vi "Read_data_from_saved_exp.vi"(10 "Path of file":path) -> (0 "Comments":string, 1 "Time Delays":dbl[](array[numeric]), 2 "Wavelengths":dbl[](array[numeric]), 3 "Data":dbl[][](array[numeric]), 4 "data raw":i32[][][][](array[numeric]), 5 "Number of points":i32, 6 "Step":dbl, 7 "Zero time delay":dbl, 8 "error out":errorcluster)   [LabVIEW 2015]
uses:
  <vilib>/Utility/file.llb/Read Delimited Spreadsheet (DBL).vi
  <vilib>/zip/NI_Unzip.lvlib
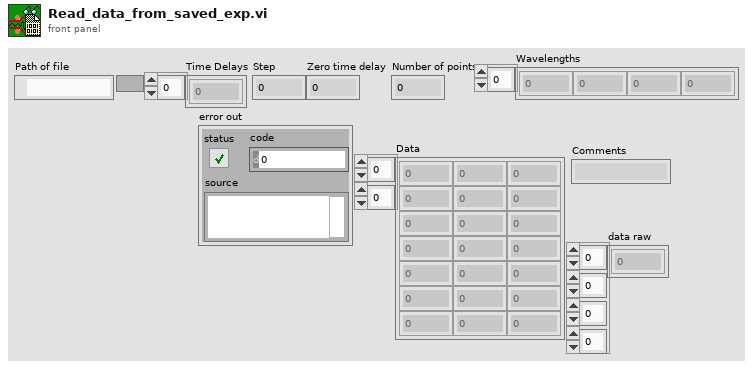
[diagram p1: front panel]
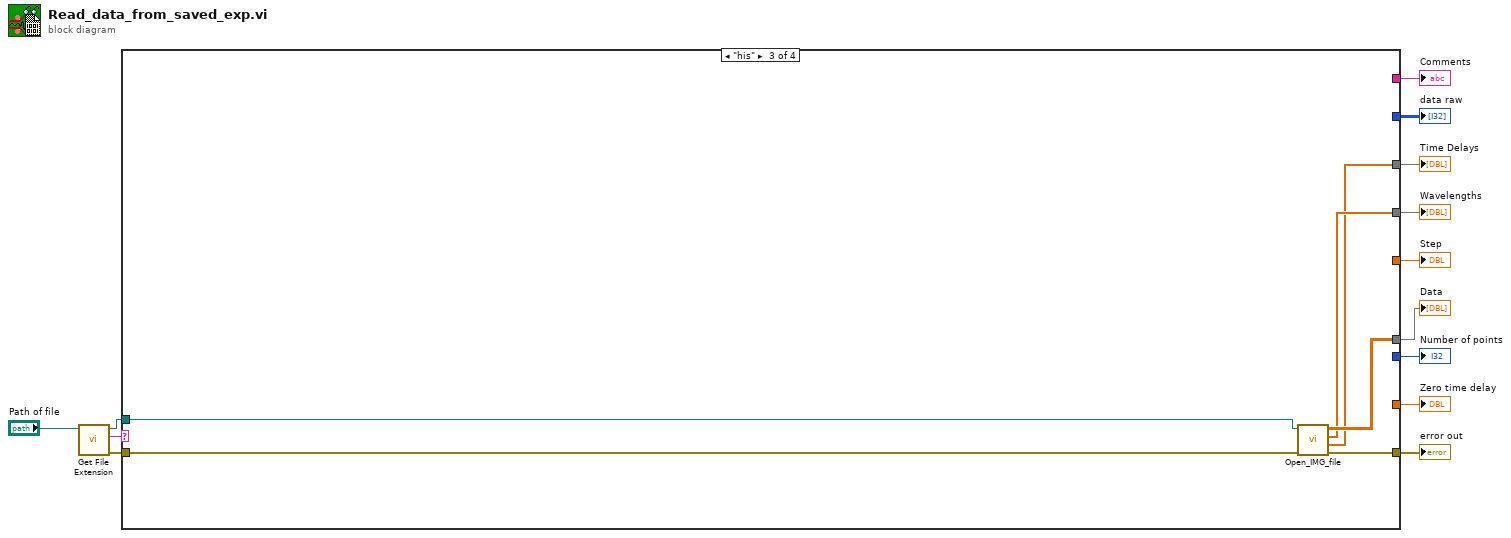
[diagram p0: block diagram]
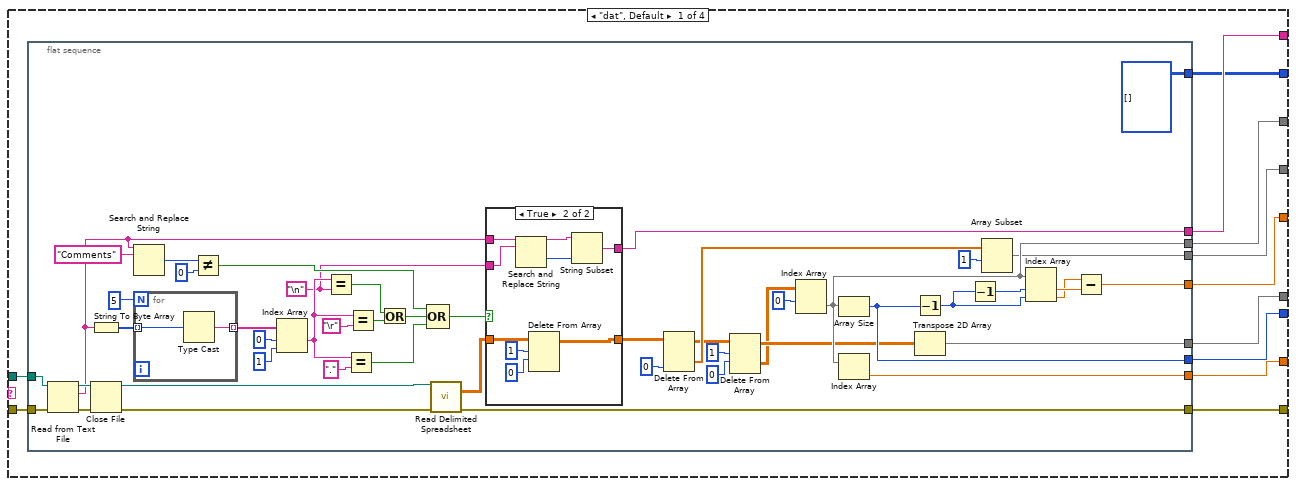
[diagram p2: hidden frame]
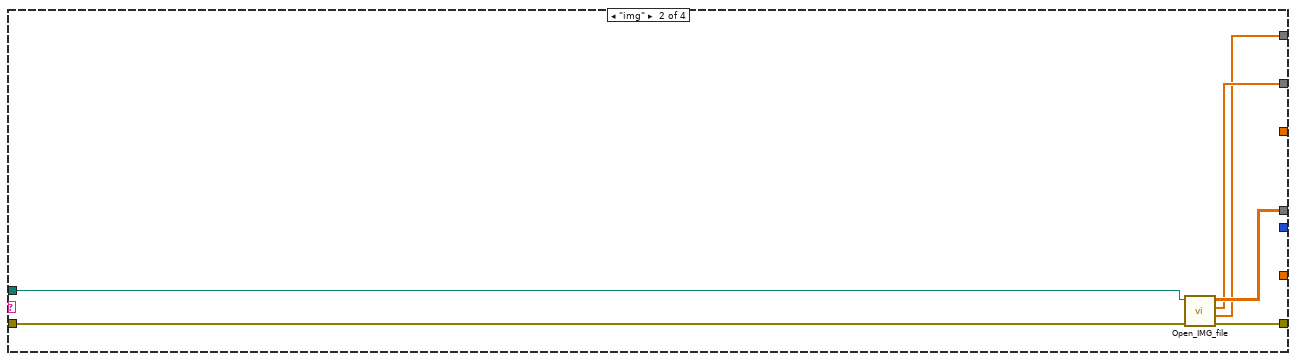
[diagram p4: hidden frame]
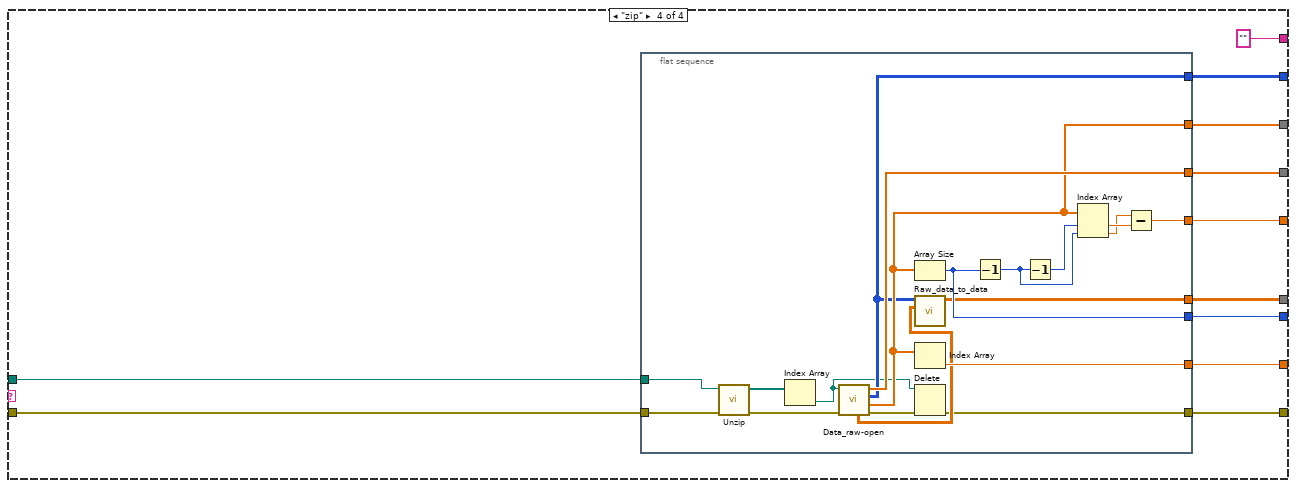
[diagram p5: hidden frame]
diagram:
  n1 = call <vilib>:"Get File Extension.vi"("file"="Path of file") -> ("error out"=w3:errorcluster, "lowercase file extension"=w4:string, "dup file"=w6:path)  [unwired: 6 in, 2 out]
  n2 = case shown="\"his\"" w4 {
    tunnel: [w24 _ _ w108] -> w13
    tunnel: [w23 w88 w94 w107] -> w12
    tunnel: [w22 w86 w92 w106] -> w11
    tunnel: [w21 _ _ w105] -> w10
    tunnel: [w20 _ _ w104] -> w9
    tunnel: [w19 w87 w93 w103] -> w8
    tunnel: w6 -> [w18 w91 w97 w102]
    tunnel: [w17 _ _ "" ("result string")] -> w5
    tunnel: w3 -> [w16 w90 w96 w101]
    tunnel: [w15 _ _ w99] -> w2
    tunnel: [w14 w89 w95 w98] -> w1
    frame "dat", Default {
      n3 = flat-sequence {
        tunnel: [w73] -> w24
        tunnel: [w72] -> w23
        tunnel: [w71] -> w22
        tunnel: w18 -> [w55]
        tunnel: [w70] -> w21
        tunnel: [w69] -> w20
        tunnel: [w68] -> w19
        tunnel: [w28] -> w17
        tunnel: w16 -> [w27]
        tunnel: [i32[][][][] [] ("data value")] -> w15
        tunnel: [w25] -> w14
        frame #0 {
          w30 = "\n"
          n4 = Read from Text File(file (use dialog)=w55, error in=w27) -> (refnum out=w54:refnum<file>, text=w31:string, error out=w52:errorcluster)  [unwired: 2 in, 1 out]
          n5 = String To Byte Array(string=w31) -> (unsigned byte array=w47:u8[])
          n6 = Close File(refnum=w54, error in=w52) -> (path=w53:path, error out=w29:errorcluster)
          n7 = Search and Replace String(input string=w31, search string="Comments") -> (number of replacements=w50:i32)  [unwired: 6 in, 3 out]
          n8 = for {
            N: 5 -> [_]
            tunnel: w47 -> [w85] mode=indexing
            tunnel: [w84] -> w45 mode=indexing
            n9 = Type Cast(x=w85) -> (*(type *) &x=w84:string)  [unwired: 1 in]
          }
          n10 = Not Equal?(x=w50, y=0) -> (x != y?=w48:bool)
          n11 = Index Array(array=w45, index #1=0 ("index"), index #2=1 ("index")) -> (element #1=w38:string)  [unwired: 1 out]
          n12 = Equal?(x=w38, y=w30) -> (x = y?=w44:bool)
          n13 = Equal?(x=w38, y=".") -> (x = y?=w36:bool)
          n14 = Equal?(x=w38, y="\r") -> (x = y?=w43:bool)
          n15 = Or(x=w44, y=w43) -> (x .or. y?=w41:bool)
          n16 = Compound Arithmetic op=OR(w48, w41, w36) -> (w35:bool)
          n17 = call-poly <vilib>:"Read Delimited Spreadsheet.vi"("file path (dialog if empty)"=w53, "error in (no error)"=w29) -> ("all rows"=w33:dbl[][], "error out"=w25:errorcluster)  [unwired: 8 in, 4 out]
          n18 = case shown="True" w35 {
            tunnel: w33 -> [w74 w83]
            tunnel: [w74 w80] -> w32
            tunnel: w31 -> [_ w78]
            tunnel: [_ w77] -> w28
            tunnel: w30 -> [_ w76]
            frame False {
            }
            frame True {
              n19 = Search and Replace String(input string=w78, search string=w76) -> (result string=w79:string, offset past replacement=w75:i32)  [unwired: 6 in, 2 out]
              n20 = Delete From Array(array=w83, length=1, index (row)=0) -> (array with subset deleted=w80:dbl[][])  [unwired: 1 in, 1 out]
              n21 = String Subset(string=w79, length (rest)=w75) -> (substring=w77:string)  [unwired: 1 in]
            }
          }
          n22 = Delete From Array(array=w32, index (col)=0 ("disabled index (col)")) -> (deleted portion=w56:dbl[], array with subset deleted=w34:dbl[][])  [unwired: 2 in]
          n23 = Delete From Array(array=w34, length=1, index (row)=0) -> (deleted portion=w65:dbl[][], array with subset deleted=w66:dbl[][])  [unwired: 1 in]
          n24 = Index Array(array=w65, index (row)=0) -> (element=w71:dbl[])  [unwired: 1 in]
          n25 = Array Size(array=w71) -> (size(s)=w73:i32)
          n26 = Index Array(array=w71) -> (element=w69:dbl)  [unwired: 1 in]
          n27 = Decrement(x=w73) -> (x-1=w60:i32)
          n28 = Transpose 2D Array(2D array=w66) -> (transposed array=w72:dbl[][])
          n29 = Decrement(x=w60) -> (x-1=w61:i32)
          n30 = Array Subset(array=w56, index=1) -> (w68:dbl[])  [unwired: 1 in]
          n31 = Index Array(array=w71, index #1=w61, index #2=w60) -> (element #1=w63:dbl, element #2=w62:dbl)
          n32 = Subtract(x=w62, y=w63) -> (x-y=w70:dbl)
        }
      }
    }
    frame "img" {
      n33 = call "Open_IMG_file.vi"("error in"=w90, "path"=w91) -> ("error out"=w89:errorcluster, "Y"=w86:dbl[], "X"=w87:dbl[], "DATA"=w88:dbl[][])  [unwired: 5 in, 1 out]
    }
    frame "his" {
      n34 = call "Open_IMG_file.vi"("error in"=w96, "path"=w97) -> ("error out"=w95:errorcluster, "Y"=w92:dbl[], "X"=w93:dbl[], "DATA"=w94:dbl[][])  [unwired: 5 in, 1 out]
    }
    frame "zip" {
      n35 = flat-sequence {
        tunnel: [w127] -> w108
        tunnel: [w111] -> w107
        tunnel: [w115] -> w106
        tunnel: w102 -> [w120]
        tunnel: [w126] -> w105
        tunnel: [w125] -> w104
        tunnel: [w116] -> w103
        tunnel: w101 -> [w119]
        tunnel: [w114] -> w99
        tunnel: [w109] -> w98
        frame #0 {
          n36 = call <vilib>:"Unzip.vi"("error in (no error)"=w119, "Zip file"=w120) -> ("error out"=w117:errorcluster, "Unzipped files"=w118:path[])  [unwired: 7 in, 1 out]
          n37 = Index Array(array=w118) -> (element=w112:path)  [unwired: 1 in]
          n38 = call "Data_raw-open.vi"("error in"=w117, "file (use dialog)"=w112) -> ("error out"=w113:errorcluster, "timedelays"=w115:dbl[], "Raw data"=w114:i32[][][][], "waves"=w116:dbl[], "Trabs precalc"=w110:dbl[][])  [unwired: 5 in]
          n39 = Array Size(array=w115) -> (size(s)=w127:i32)
          n40 = call "Raw_data_to_data.vi"("Trabs precalc"=w110, "Raw data"=w114) -> ("Exp data"=w111:dbl[][])  [unwired: 9 in]
          n41 = Index Array(array=w115) -> (element=w125:dbl)  [unwired: 1 in]
          n42 = Delete(path (use dialog)=w112, error in=w113) -> (error out=w109:errorcluster)  [unwired: 3 in, 2 out]
          n43 = Decrement(x=w127) -> (x-1=w121:i32)
          n44 = Decrement(x=w121) -> (x-1=w122:i32)
          n45 = Index Array(array=w115, index #1=w122, index #2=w121) -> (element #1=w124:dbl, element #2=w123:dbl)
          n46 = Subtract(x=w123, y=w124) -> (x-y=w126:dbl)
        }
      }
    }
  }
  "Number of points" <- w13
  "Data" <- w12
  "Time Delays" <- w11
  "Step" <- w10
  "Zero time delay" <- w9
  "Wavelengths" <- w8
  "Comments" <- w5
  "data raw" <- w2
  "error out" <- w1
